vi "Finish.vi"   [LabVIEW 2016]
doc: "This VI is called just before exiting. It is expected to close I/O refnum, save collected data, etc."
uses:
  <vilib>/Rock Robotics/WPI/Utilities/WPI_GetSetVariantRefNum.vi
types:
  T1 = typedef "WPI_RelayDevRef.ctl" = cluster{"DevStatus":errorcluster, "Relay Channel":T2, "Relay Direction":T3}
  T2 = typedef "FPGA_DIORelayChannel.ctl" = enum8{"Relay 0", "Relay 1", "Relay 2", "Relay 3", "Invalid"}
  T3 = typedef "WPI_RelayDirection.ctl" = enum16{"Both directions", "Forward only", "Reverse only"}
  T4 = typedef "WPI_ServoDeviceRef.ctl" = cluster{"DeviceStatus":errorcluster, "PWM Channel":T5, "DeadBand":T6}
  T5 = typedef "FPGA_DIOPWMChannel.ctl" = enum8{"PWM 0", "PWM 1", "PWM 2", "PWM 3", "PWM 4", "PWM 5", "PWM 6", "PWM 7", "PWM 8", "PWM 9", "PWM MXP 0", "PWM MXP 1", "PWM MXP 2", "PWM MXP 3", "PWM MXP 4", "PWM MXP 5", "PWM MXP 6", "PWM MXP 7", "PWM MXP 8", "PWM MXP 9", "Invalid"}
  T6 = typedef "WPI_PWMDeadband.ctl" = cluster{"Name":string, "maxPositivePwm":i32, "minPositivePwm":i32, "centerPwm":i32, "maxNegativePwm":i32, "minNegativePwm":i32, "angularRange":u16}
  T7 = typedef "WPI_AccelerometerDevRef.ctl" = cluster{"DevStatus":errorcluster, "Scaling":T8, "Analog Channels":T9, "I2C Bus":T11, "SPI Bus":T12, "Accel Range":T13, "ADXL Axes":T14, "Handle":i32, "Device Address":u8, "Accel Type":enum16{"Analog", "ADXL345 I2C", "ADXL345 SPI", "Internal", "ADXL362 SPI"}}
  T8 = typedef "WPI_AccelerometerScaling.ctl" = cluster{"Gain (VoltsPerG)":dbl, "Center Voltage":dbl}
  T9 = typedef "WPI_AccelerometerAnalogChannels.ctl" = cluster{"X-Axis":T10, "Y-Axis":T10, "Z-Axis":T10}
  T10 = typedef "FPGA_AIChannel.ctl" = enum8{"AI 0", "AI 1", "AI 2", "AI 3", "AI MXP 0", "AI MXP 1", "AI MXP 2", "AI MXP 3", "Invalid"}
  T11 = typedef "i2c_bus.ctl" = enum16{"I2C On-Board", "I2C MXP", "Invalid"}
  T12 = typedef "spi_bus.ctl" = enum16{"SPI On-Board, CS0", "SPI On-Board, CS1", "SPI On-Board, CS2", "SPI On-Board, CS3", "SPI MXP", "Invalid"}
  T13 = typedef "ADXL345 Range.ctl" = u8
  T14 = typedef "WPI_AccelerometerADXL345 Axes.ctl" = cluster{"X-Axis":bool, "Y-Axis":bool, "Z-Axis":bool}
  T15 = typedef "WPI_EncoderDevRef.ctl" = cluster{"DevStatus":errorcluster, "EncoderIndex":T16, "CounterIndex":T17, "DistancePerCount":dbl, "Decoding Type":T18}
  T16 = typedef "FPGA_EncoderIdx.ctl" = enum8{"Enc 0", "Enc 1", "Enc 2", "Enc 3", "Enc 4", "Enc 5", "Enc 6", "Enc 7", "Invalid"}
  T17 = typedef "FPGA_CounterCtrSystemIndex.ctl" = enum8{"Ctr 0", "Ctr 1", "Ctr 2", "Ctr 3", "Ctr 4", "Ctr 5", "Ctr 6", "Ctr 7", "Invalid"}
  T18 = typedef "WPI_EncoderType.ctl" = enum16{"1x", "2x", "4x"}
  T19 = typedef "WPI_GyroDevRef.ctl" = cluster{"DevStatus":errorcluster, "Analog Channel":T10, "Offset":dbl, "Gain (VoltsPerDegree/Second)":dbl, "Gyro Type":enum16{"Analog", "XRS450"}, "Handle":i32, "SPI Bus":T12, "Device Found":bool, "Sample Rate":dbl, "Calibrate On Open":bool}
  T20 = typedef "WPI_JoystickDevRef.ctl" = cluster{"Device":T21}
  T21 = typedef "WPI_JoystickDeviceEnum.ctl" = enum16{"USB 0", "USB 1", "USB 2", "USB 3", "USB 4", "USB 5"}
  T22 = typedef "WPI_RobotDriveDevRef.ctl" = cluster{"DevStatus":errorcluster, "Motors[]":T23[], "Square Inputs":bool, "Max Output":dbl}
  T23 = typedef "WPI_MotorControlDeviceRef.ctl" = cluster{"DeviceStatus":errorcluster, "Type":T24, "PWM":cluster{"PWM Channel":T5, "DeadBand":T6}, "CAN":cluster{"Device Number":u8, "SetOutput VI Ref":variant, "GetOutput VI Ref":variant, "Enable VI Ref":variant, "Disable VI Ref":variant, "Data":variant}, "Invert":bool}
  T24 = typedef "WPI_MotorControlType.ctl" = enum16{"PWM", "CAN"}
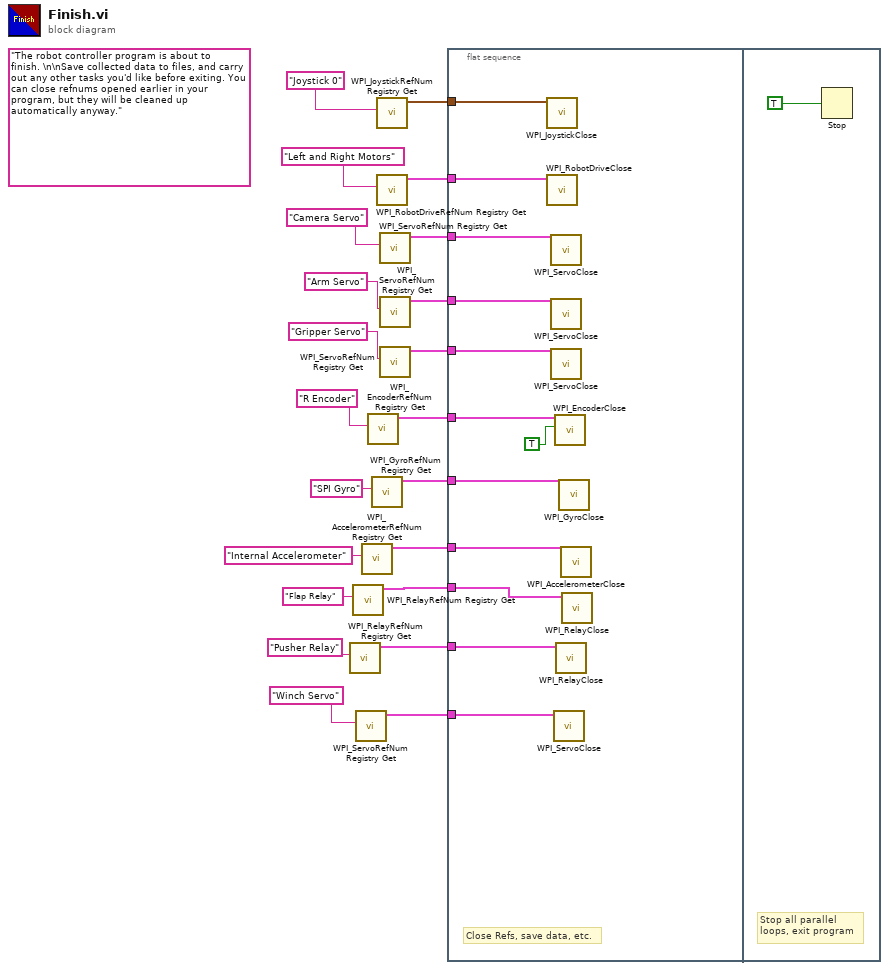
[diagram p0: block diagram]
diagram:
  (unwired) "The robot controller program is about to finish. \n\nSave collected data to files, and carry out any other tasks you'd like before exiting. You can close refnums opened earlier in your program, but they will be cleaned up automatically anyway."
  n1 = call <vilib>:"WPI_RelayRefNum Registry Get.vi"("refnum name"="Pusher Relay") -> ("RelayDevRef"=w3:T1)  [unwired: 9 in, 1 out]
  n2 = call <vilib>:"WPI_RelayRefNum Registry Get.vi"("refnum name"="Flap Relay") -> ("RelayDevRef"=w5:T1)  [unwired: 9 in, 1 out]
  n3 = call <vilib>:"WPI_ServoRefNum Registry Get.vi"("refnum name"="Winch Servo") -> ("ServoDeviceRef"=w1:T4)  [unwired: 9 in, 1 out]
  n4 = call <vilib>:"WPI_AccelerometerRefNum Registry Get.vi"("refnum name"="Internal Accelerometer") -> ("AccelerometerDevRef"=w10:T7)  [unwired: 9 in, 1 out]
  n5 = call <vilib>:"WPI_EncoderRefNum Registry Get.vi"("refnum name"="R Encoder") -> ("EncoderDevRef"=w11:T15)  [unwired: 9 in, 1 out]
  n6 = call <vilib>:"WPI_GyroRefNum Registry Get.vi"("refnum name"="SPI Gyro") -> ("GyroDevRef"=w9:T19)  [unwired: 9 in, 1 out]
  n7 = call <vilib>:"WPI_JoystickRefNum Registry Get.vi"("refnum name"="Joystick 0") -> ("JoystickDevRef"=w19:T20)  [unwired: 1 in, 9 out]
  n8 = call <vilib>:"WPI_RobotDriveRefNum Registry Get.vi"("refnum name"="Left and Right Motors") -> ("RobotDriveDevRef"=w20:T22)  [unwired: 1 in, 9 out]
  n9 = call <vilib>:"WPI_ServoRefNum Registry Get.vi"("refnum name"="Camera Servo") -> ("ServoDeviceRef"=w17:T4)  [unwired: 9 in, 1 out]
  n10 = call <vilib>:"WPI_ServoRefNum Registry Get.vi"("refnum name"="Arm Servo") -> ("ServoDeviceRef"=w16:T4)  [unwired: 9 in, 1 out]
  n11 = call <vilib>:"WPI_ServoRefNum Registry Get.vi"("refnum name"="Gripper Servo") -> ("ServoDeviceRef"=w14:T4)  [unwired: 9 in, 1 out]
  n12 = flat-sequence {
    tunnel: w20 -> [w34]
    tunnel: w19 -> [w33]
    tunnel: w17 -> [w32]
    tunnel: w16 -> [w31]
    tunnel: w14 -> [w30]
    tunnel: w11 -> [w28]
    tunnel: w10 -> [w27]
    tunnel: w9 -> [w26]
    tunnel: w5 -> [w25]
    tunnel: w3 -> [w24]
    tunnel: w1 -> [w23]
    frame #0 {
      # "Close Refs, save data, etc."
      n13 = call <vilib>:"WPI_JoystickClose.vi"("JoystickDevRef"=w33) -> ()  [unwired: 11 out]
      n14 = call <vilib>:"WPI_RobotDriveClose.vi"("RobotDriveDevRef"=w34) -> ()  [unwired: 1 in, 10 out]
      n15 = call <vilib>:"WPI_ServoClose.vi"("ServoDeviceRef"=w32) -> ()  [unwired: 10 in, 1 out]
      n16 = call <vilib>:"WPI_ServoClose.vi"("ServoDeviceRef"=w31) -> ()  [unwired: 10 in, 1 out]
      n17 = call <vilib>:"WPI_ServoClose.vi"("ServoDeviceRef"=w30) -> ()  [unwired: 10 in, 1 out]
      n18 = call <vilib>:"WPI_ServoClose.vi"("ServoDeviceRef"=w23) -> ()  [unwired: 10 in, 1 out]
      n19 = call <vilib>:"WPI_EncoderClose.vi"("Close Dependencies"=TRUE, "EncoderDevRef"=w28) -> ()  [unwired: 9 in, 1 out]
      n20 = call <vilib>:"WPI_RelayClose.vi"("RelayDevRef"=w24) -> ()  [unwired: 10 in, 1 out]
      n21 = call <vilib>:"WPI_GyroClose.vi"("GyroDevRef"=w26) -> ()  [unwired: 10 in, 1 out]
      n22 = call <vilib>:"WPI_AccelerometerClose.vi"("AccelerometerDevRef"=w27) -> ()  [unwired: 10 in, 1 out]
      n23 = call <vilib>:"WPI_RelayClose.vi"("RelayDevRef"=w25) -> ()  [unwired: 10 in, 1 out]
    }
    frame #1 {
      # "Stop all parallel\nloops, exit program"
      n24 = Stop(stop? (T)=TRUE ("Quit")) -> ()
    }
  }
